vi "Get TypeGUID.vi"(8 "error in (no error)":errorcluster caption="错误输入（无错误）", 11 "Section输入":refnum<class "Section.lvclass">) -> (0 "error out":errorcluster caption="错误输出", 2 "TypeGUID":string, 3 "Section输出":refnum<class "Section.lvclass">)   [LabVIEW 2013]
uses:
  Section.lvclass
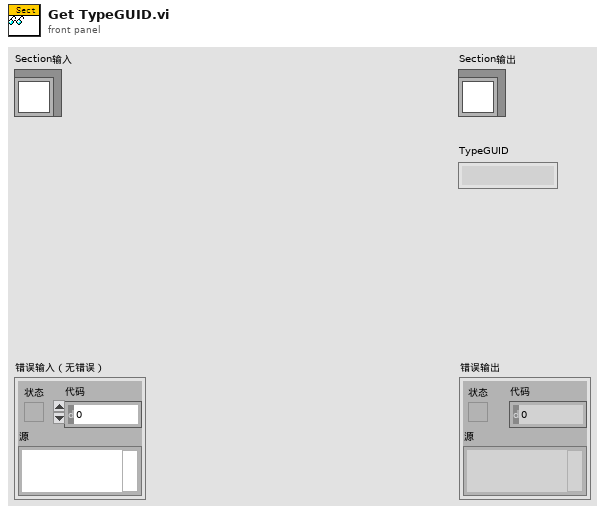
[diagram p1: front panel]
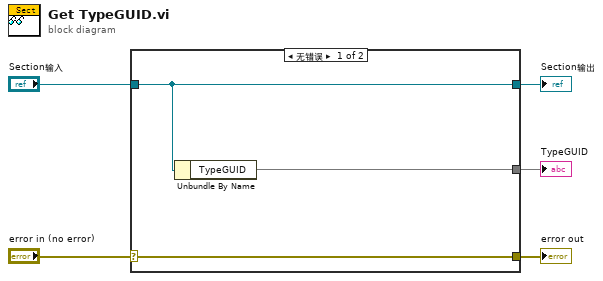
[diagram p0: block diagram]
diagram:
  n1 = case shown="无错误" "error in (no error)" {
    selector: "error in (no error)" -> [w8 w9]
    tunnel: [w8 w9] -> w4
    tunnel: [w7 w10] -> w2
    tunnel: "Section输入" -> [w7 w10]
    tunnel: [w6 _] -> w1
    frame No Error {
      n2 = Unbundle By Name(w7) -> ("TypeGUID"=w6)
    }
    frame Error {
    }
  }
  "error out" <- w4
  "Section输出" <- w2
  "TypeGUID" <- w1
